vi "ConvertErrToString.vi"(0 "error in (no error)":errorcluster) -> (1 "String":string, 2 "color":string)   [LabVIEW 2015]
uses:
  vi.lib/Utility/error.llb/DialogType.ctl
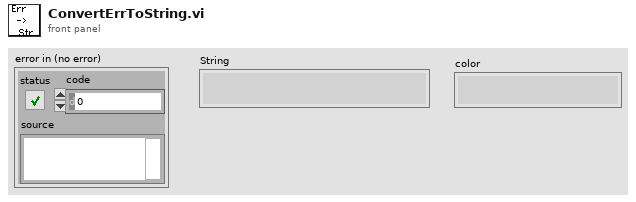
[diagram p1: front panel]
types:
  T1 = typedef "DialogType.ctl" = u16
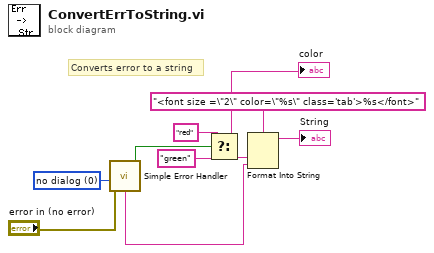
[diagram p0: block diagram]
diagram:
  w4 = T1 0 items=["no dialog", "OK message", "continue or stop message", "OK message + warnings", "continue/stop + warnings"] ("type of dialog (OK msg:1)")
  # "Converts error to a string"
  n1 = call "Simple Error Handler.vi"("type of dialog (OK msg:1)"=w4, "error in (no error)"="error in (no error)") -> ("error?"=w1:bool, "message"=w2:string)  [unwired: 3 in, 3 out]
  n2 = Select(t="red" ("format string"), s=w1, f="green" ("format string")) -> (s? t:f=w8:string)
  "color" <- w8
  n3 = Format Into String(format string="<font size =\"2\" color=\"%s\" class='tab'>%s</font>", w8, w2) -> (resulting string=→"String":string)  [unwired: 2 in, 1 out]
